vi "SR830DSP_RS232_NSOM.vi"(0 "Lecturas":i32=10, 1 "delay before read (ms)":u32=100) -> (2 "X promedio":dbl, 3 "Y promedio":dbl, 4 "X's":dbl[](array[numeric]), 5 "Y's":dbl[](array[numeric]))   [LabVIEW 2018]
doc: "This example performs a serial port write and a serial port read. The parameters set for the serial port must match the parameters of the connected instrument or device. The VISA Configure Serial Port VI sets the configuration parameters. The front panel displays the controls used to configure the basic parameters, such as baud rate, data bits, and parity. The VI passes the VISA resource name to other VIs that perform operations on that VISA resource. The VISA Write function sends a command to the serial device and the VISA Read function returns data based on the command. The VISA Close function then closes the reference to the serial device. It is important to close the reference; otherwise, further communication through that port might not be possible."
uses:
  Serial - Settings.ctl
  <vilib>/Analysis/baseanly.llb/Mean (DBL).vi
  <vilib>/Instr/_visa.llb/VISA Configure Serial Port (Instr).vi
  <vilib>/Analysis/NI_AALBase.lvlib
panel:
  out "Y":string
  out "X":string
  in  "Serial Settings":T1={"baud rate"=9600, "data bits"=8, "parity"=enum."None", "stop bits"=10, "flow control"=0} {"flow control" items=["None"=0, "XON/XOFF"=1, "RTS/CTS"=2, "DTR/DSR"=4]; "stop bits" items=["1.0"=10, "1.5"=15, "2.0"=20]; "data bits" min=5 max=8 step=1; "baud rate" items=["75"=75, "110"=110, "134"=134, "150"=150, "300"=300, "600"=600, "1200"=1200, "1800"=1800, "2400"=2400, "4800"=4800, "7200"=7200, "9600"=9600, "14400"=14400, "19200"=19200, "28800"=28800, "38400"=38400, "56000"=56000, "57600"=57600, "115200"=115200, "128000"=128000, "230400"=230400]}
  in  "VISA resource name":refnum<visa-resource-name>="COM3"
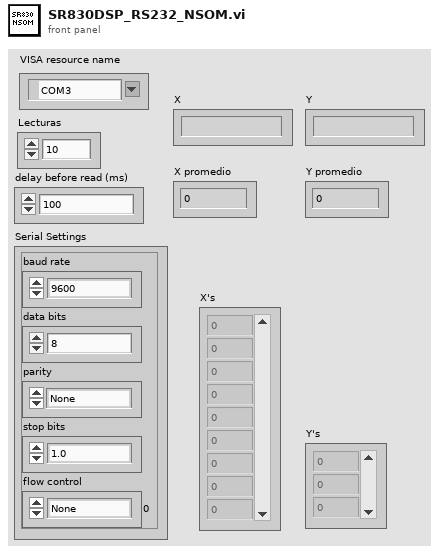
[diagram p1: front panel]
types:
  T1 = typedef "Serial - Settings.ctl" = cluster{"baud rate":u32, "data bits":u16, "parity":enum16{"None", "Odd", "Even", "Mark", "Space"}, "stop bits":u16, "flow control":u16}
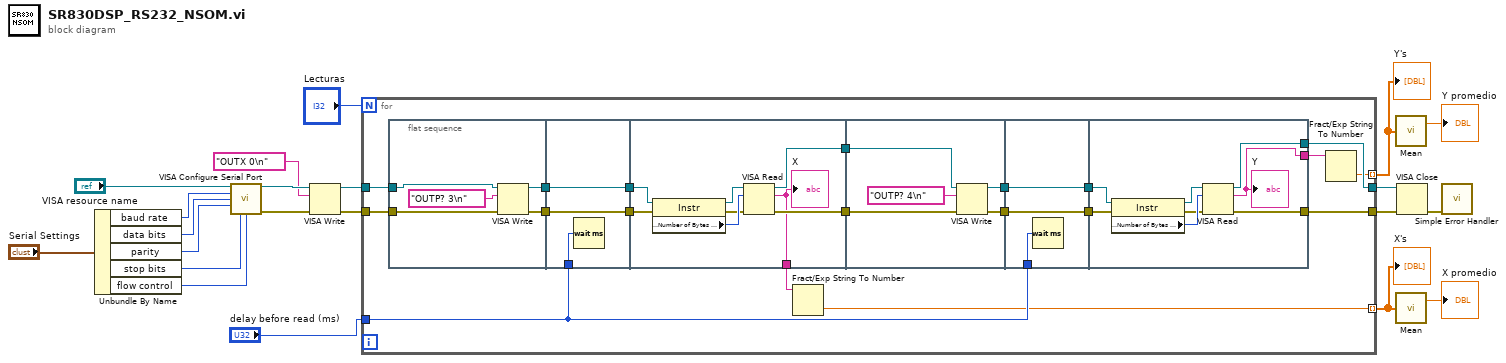
[diagram p0: block diagram]
diagram:
  n1 = Unbundle By Name("Serial Settings") -> ("baud rate"=w15:u32, "data bits"=w14:u16, "parity"=w13:enum16{"None", "Odd", "Even", "Mark", "Space"}, "stop bits"=w12:u16, "flow control"=w11:u16)
  n2 = call-poly "VISA Configure Serial Port"("VISA resource name"="VISA resource name", "baud rate (9600)"=w15, "data bits (8)"=w14, "parity (0:none)"=w13, "stop bits (10: 1 bit)"=w12, "flow control (0:none)"=w11) -> ("VISA resource name out"=w19:refnum<visa-resource-name>, "error out"=w20:errorcluster)  [unwired: 3 in, 5 out]
  n3 = VISA Write(VISA resource name=w19, write buffer="OUTX 0\n" ("Command"), error in (no error)=w20) -> (VISA resource name out=w7:refnum<visa-resource-name>, error out=w6:errorcluster)  [unwired: 1 out]
  n4 = for {
    N: "Lecturas" -> [_]
    tunnel: "delay before read (ms)" -> [w40]
    tunnel: w7 -> [w39]
    tunnel: [w26] -> w8
    tunnel: w6 -> [w38]
    tunnel: [w27] -> w5
    tunnel: [w24] -> w3 mode=indexing
    tunnel: [w22] -> w4 mode=indexing
    n5 = flat-sequence {
      tunnel: w39 -> [w44]
      tunnel: w38 -> [w43]
      tunnel: [w42] -> w37
      tunnel: [w41] -> w34
      tunnel: w40 -> [w48]
      tunnel: w37 -> [w47]
      tunnel: [w47] -> w36
      tunnel: [w46] -> w35
      tunnel: w34 -> [w46]
      tunnel: w36 -> [w53]
      tunnel: w35 -> [w52]
      tunnel: [w51] -> w29
      tunnel: [w50] -> w28
      tunnel: [w49] -> w25
      tunnel: [w60] -> w32
      tunnel: [w59] -> w30
      tunnel: w29 -> [w58]
      tunnel: w28 -> [w57]
      tunnel: w40 -> [w64]
      tunnel: [w63] -> w33
      tunnel: w32 -> [w63]
      tunnel: [w62] -> w31
      tunnel: w30 -> [w62]
      tunnel: w33 -> [w69]
      tunnel: w31 -> [w68]
      tunnel: [w67] -> w27
      tunnel: [w66] -> w26
      tunnel: [w65] -> w23
      frame #0 {
        n6 = VISA Write(VISA resource name=w44, write buffer="OUTP? 3\n" ("Command"), error in (no error)=w43) -> (VISA resource name out=w42:refnum<visa-resource-name>, error out=w41:errorcluster)  [unwired: 1 out]
      }
      frame #1 {
        n7 = Wait (ms)(milliseconds to wait=w48) -> ()  [unwired: 1 out]
      }
      frame #2 {
        n8 = property class="Instr"(reference=w53, error in=w52) -> (reference out=w54:refnum<visa-resource-name>, error out=w55:errorcluster, "Serial Settings:Number of Bytes at Serial Port"=w56:u32)
        n9 = VISA Read(VISA resource name=w54, byte count=w56, error in (no error)=w55) -> (VISA resource name out=w50:refnum<visa-resource-name>, read buffer=w49:string, error out=w51:errorcluster)  [unwired: 1 out]
        "X" <- w49
      }
      frame #3 {
        n10 = VISA Write(VISA resource name=w57, write buffer="OUTP? 4\n" ("Command"), error in (no error)=w58) -> (VISA resource name out=w60:refnum<visa-resource-name>, error out=w59:errorcluster)  [unwired: 1 out]
      }
      frame #4 {
        n11 = Wait (ms)(milliseconds to wait=w64) -> ()  [unwired: 1 out]
      }
      frame #5 {
        n12 = property class="Instr"(reference=w69, error in=w68) -> (reference out=w70:refnum<visa-resource-name>, error out=w71:errorcluster, "Serial Settings:Number of Bytes at Serial Port"=w72:u32)
        n13 = VISA Read(VISA resource name=w70, byte count=w72, error in (no error)=w71) -> (VISA resource name out=w67:refnum<visa-resource-name>, read buffer=w65:string, error out=w66:errorcluster)  [unwired: 1 out]
        "Y" <- w65
      }
    }
    n14 = Fract/Exp String To Number(string=w25) -> (number=w24:dbl)  [unwired: 3 in, 1 out]
    n15 = Fract/Exp String To Number(string=w23) -> (number=w22:dbl)  [unwired: 3 in, 1 out]
  }
  "X's" <- w3
  "Y's" <- w4
  n16 = call-poly <vilib>:"Mean.vi"("X"=w4) -> ("mean"=→"Y promedio":dbl)  [unwired: 1 out]
  n17 = call-poly <vilib>:"Mean.vi"("X"=w3) -> ("mean"=→"X promedio":dbl)  [unwired: 1 out]
  n18 = VISA Close(VISA resource name=w5, error in (no error)=w8) -> (error out=w18:errorcluster)
  n19 = call <vilib>:"Simple Error Handler.vi"("error in (no error)"=w18) -> ()  [unwired: 1 in, 8 out]
